vi "NumArrayToHexStrArr.vi"(1 "Array of numbers":i32[](array[numeric])) -> (0 "concatenated string":string)   [LabVIEW 2017]
panel:
  out "spreadsheet string":string
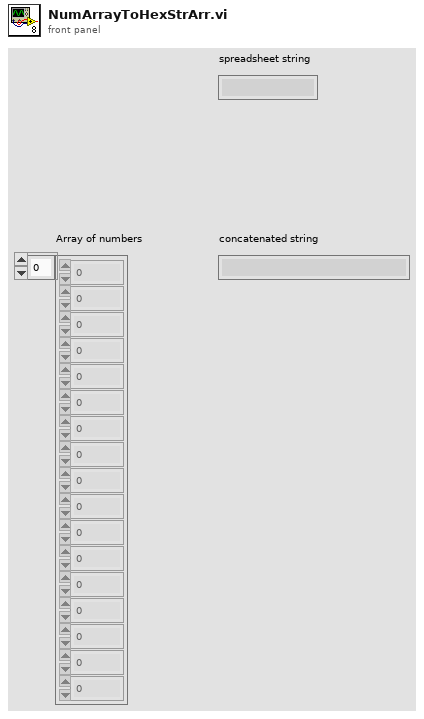
[diagram p1: front panel]
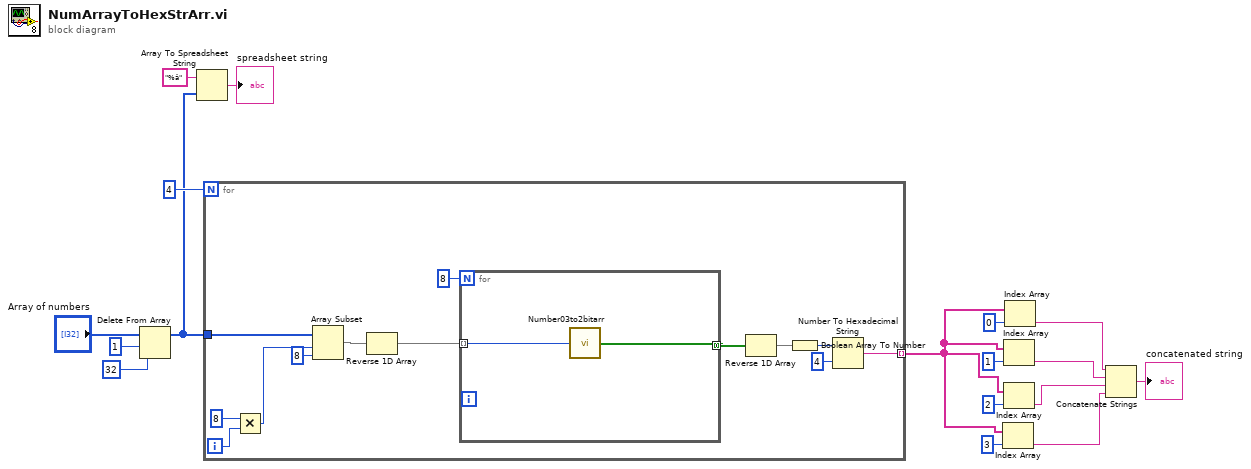
[diagram p0: block diagram]
diagram:
  n1 = Delete From Array(array="Array of numbers", length=1, index=32) -> (array with subset deleted=w3:i32[])  [unwired: 1 out]
  n2 = Array To Spreadsheet String(array=w3, 3:"%â" ("format string")) -> (spreadsheet string=→"spreadsheet string":string)  [unwired: 1 in]
  n3 = for {
    N: 4 -> [_]
    tunnel: w3 -> [w22]
    tunnel: [w24] -> w10 mode=indexing
    i -> [w30]
    n4 = Multiply(x=8, y=w30) -> (x*y=w21:i32)
    n5 = Array Subset(array=w22, index=w21, length=8) -> (w19:i32[])
    n6 = Reverse 1D Array(array=w19) -> (reversed array=w18:i32[])
    n7 = for {
      N: 8 -> [_]
      tunnel: w18 -> [w31] mode=indexing
      tunnel: [w32] -> w26 mode=concatenating
      n8 = call "Number03to2bitarr.vi"("Value 0-3"=w31) -> ("2 bit array"=w32:bool[])
    }
    n9 = Reverse 1D Array(array=w26) -> (reversed array=w25:bool[])
    n10 = Boolean Array To Number(Boolean array=w25) -> (number=w27:u32)
    n11 = Number To Hexadecimal String(1:i16 4 ("width (-)"), 2:w27) -> (0:w24:string)
  }
  n12 = Index Array(array=w10, index=3) -> (element=w6:string)
  n13 = Index Array(array=w10, index=1) -> (element=w8:string)
  n14 = Index Array(array=w10, index=2) -> (element=w7:string)
  n15 = Index Array(array=w10, index=0) -> (element=w9:string)
  n16 = Concatenate Strings(w9, w8, w7, w6) -> (→"concatenated string":string)
